vi "what key was pressed (SubVI).vi"(11 "keys pressed":T1(array[ring])) -> (0 "D":bool, 1 "A":bool, 2 "Left":bool, 3 "Right":bool)   [LabVIEW 2018]
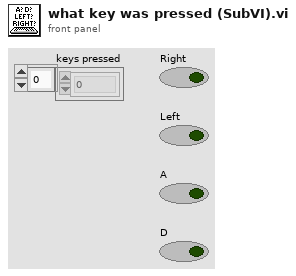
[diagram p1: front panel]
types:
  T1 = enum16{"0", "1", "2", "3", "4", "5", "6", "7", "8", "9", "A", "B", "C", "D", "E", "F", "G", "H", "I", "J", "K", "L", "M", "N", "O", "P", "Q", "R", "S", "T", "U", "V", "W", "X", "Y", "Z", "F1", "F2", "F3", "F4", "F5", "F6", "F7", "F8", "F9", "F10", "F11", "F12", "F13", "F14", "F15", "ADD", "BACK", "BACKSLASH", "CAPITAL", "COMMA", "DECIMAL", "DELETE", "DIVIDE", "DOWN", "END", "EQUALS", "ESCAPE", "GRAVE (`)", "HOME", "INSERT", "LBRACKET", "LCONTROL", "LEFT", "L ALT", "LSHIFT", "LWIN", "MINUS", "MULTIPLY", "NEXT", "NUMLOCK", "NUMPAD_0", "NUMPAD_1", "NUMPAD_2", "NUMPAD_3", "NUMPAD_4", "NUMPAD_5", "NUMPAD_6", "NUMPAD_7", "NUMPAD_8", "NUMPAD_9", "PAUSE", "PERIOD", "PRIOR (PG UP)", "RBRACKET", "RCONTROL", "RETURN", "RIGHT", "R ALT", "RSHIFT", "RWIN", "SCROLL", "SEMICOLON", "SLASH", "SPACE", "SUBTRACT", "TAB", "UP", "ENTER (num pad)", "' (quote)"}[]
  T2 = enum16{"0", "1", "2", "3", "4", "5", "6", "7", "8", "9", "A", "B", "C", "D", "E", "F", "G", "H", "I", "J", "K", "L", "M", "N", "O", "P", "Q", "R", "S", "T", "U", "V", "W", "X", "Y", "Z", "F1", "F2", "F3", "F4", "F5", "F6", "F7", "F8", "F9", "F10", "F11", "F12", "F13", "F14", "F15", "ADD", "BACK", "BACKSLASH", "CAPITAL", "COMMA", "DECIMAL", "DELETE", "DIVIDE", "DOWN", "END", "EQUALS", "ESCAPE", "GRAVE (`)", "HOME", "INSERT", "LBRACKET", "LCONTROL", "LEFT", "L ALT", "LSHIFT", "LWIN", "MINUS", "MULTIPLY", "NEXT", "NUMLOCK", "NUMPAD_0", "NUMPAD_1", "NUMPAD_2", "NUMPAD_3", "NUMPAD_4", "NUMPAD_5", "NUMPAD_6", "NUMPAD_7", "NUMPAD_8", "NUMPAD_9", "PAUSE", "PERIOD", "PRIOR (PG UP)", "RBRACKET", "RCONTROL", "RETURN", "RIGHT", "R ALT", "RSHIFT", "RWIN", "SCROLL", "SEMICOLON", "SLASH", "SPACE", "SUBTRACT", "TAB", "UP", "ENTER (num pad)", "' (quote)"}
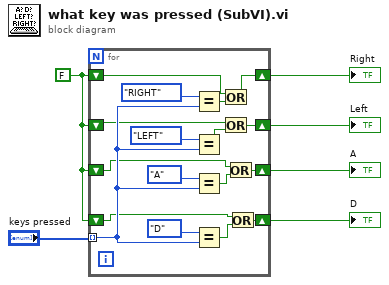
[diagram p0: block diagram]
diagram:
  w6 = FALSE
  n1 = for {
    tunnel: "keys pressed" -> [w19] mode=indexing
    shift-right: [w17] -> w2
    shift-left: w6 -> [w16]
    shift-right: [w14] -> w3
    shift-left: w6 -> [w13]
    shift-right: [w11] -> w4
    shift-left: w6 -> [w10]
    shift-right: [w8] -> w5
    shift-left: w6 -> [w7]
    n2 = Equal?(x=T2."RIGHT" ("element"), y=w19) -> (x = y?=w18:bool)
    n3 = Equal?(x=T2."LEFT" ("element"), y=w19) -> (x = y?=w15:bool)
    n4 = Equal?(x=T2."A" ("element"), y=w19) -> (x = y?=w12:bool)
    n5 = Equal?(x=T2."D" ("element"), y=w19) -> (x = y?=w9:bool)
    n6 = Or(x=w16, y=w18) -> (x .or. y?=w17:bool)
    n7 = Or(x=w13, y=w15) -> (x .or. y?=w14:bool)
    n8 = Or(x=w10, y=w12) -> (x .or. y?=w11:bool)
    n9 = Or(x=w7, y=w9) -> (x .or. y?=w8:bool)
  }
  "D" <- w5
  "A" <- w4
  "Left" <- w3
  "Right" <- w2
